vi "Write Header.vi"(6 "Delimiter":string=",", 8 "Error In":errorcluster, 11 "Log In":refnum<file>) -> (0 "Error Out":errorcluster, 3 "Log Out":refnum<file>)   [LabVIEW 2025, in "LOGlib_LV2025.lvlib" / "File.lvlib"]
uses:
  File.lvlib
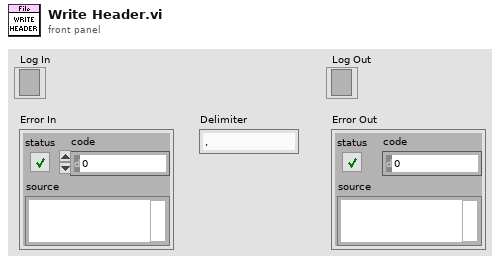
[diagram p1: front panel]
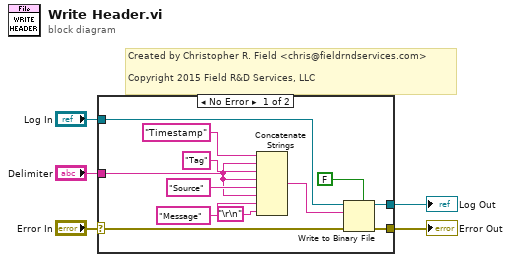
[diagram p0: block diagram]
diagram:
  # "Created by Christopher R. Field <chris@fieldrndservices.com>\n\nCopyright 2015 Field R&D Services, LLC"
  n1 = case shown="No Error" "Error In" {
    selector: "Error In" -> [w14 w18]
    tunnel: "Log In" -> [w16 w19]
    tunnel: [w15 w19] -> w4
    tunnel: [w13 w18] -> w2
    tunnel: "Delimiter" -> [w8 _]
    frame No Error {
      n2 = Concatenate Strings("Timestamp", w8, "Tag", w8, "Source", w8, "Message", "\r\n") -> (w12:string)
      n3 = Write to Binary File(file (use dialog)=w16, data=w12, error in=w14, 5:FALSE ("prepend array or string size? (T)")) -> (refnum out=w15:refnum<file>, error out=w13:errorcluster)  [unwired: 2 in, 1 out]
    }
    frame Error {
    }
  }
  "Log Out" <- w4
  "Error Out" <- w2
